vi "trackGlobVarWrite.vi"(0 "dacStepSize20Bit":i32, 1 "dacStartRegister20Bit":i32, 2 "nOfSteps":i32, 3 "nOfScans":i32, 4 "invertScan":bool, 8 "VoltOrScaler?":bool, 9 "waitForKepco(us)":u32, 11 "waitAfterReset(us)":u32 caption="waitAfterReset(25nsTicks)") -> ()   [LabVIEW 2014]
uses:
  <vilib>/rvi/Emulation/niFpgaSctlEmulationGetInTimedLoop.vi
  trackGlobVar.vi
  <vilib>/rvi/Emulation/niFpgaProcessEmulError.vi
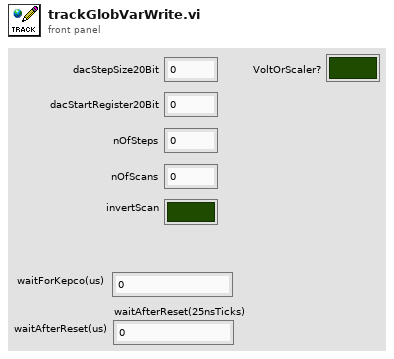
[diagram p1: front panel]
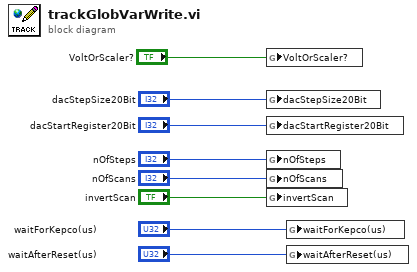
[diagram p0: block diagram]
diagram:
  n1 = global write "trackGlobVar.vi" "VoltOrScaler?"("VoltOrScaler?") -> ()
  n2 = global write "trackGlobVar.vi" "dacStepSize20Bit"("dacStepSize20Bit") -> ()
  n3 = global write "trackGlobVar.vi" "dacStartRegister20Bit"("dacStartRegister20Bit") -> ()
  n4 = global write "trackGlobVar.vi" "nOfSteps"("nOfSteps") -> ()
  n5 = global write "trackGlobVar.vi" "nOfScans"("nOfScans") -> ()
  n6 = global write "trackGlobVar.vi" "invertScan"("invertScan") -> ()
  n7 = global write "trackGlobVar.vi" "waitForKepco(us)"("waitForKepco(us)") -> ()
  n8 = global write "trackGlobVar.vi" "waitAfterReset(us)"("waitAfterReset(us)") -> ()
